vi "Digitizer Analyze_Xout FFT.vi"(7 "Pins":string[](array[string])=["Xout"], 8 "error in":errorcluster, 9 "Published Data Id":string[](array[string]), 10 "Waveform Data In":waveform(dbl)[](array[waveform])=[{"t0"=timestamp(3637030365.2340937 s since 1904-01-01), "dt"=3.3333333333333334e-08, "Y"=array[5343 elements]}, {"t0"=timestamp(3637030365.2340937 s since 1904-01-01), "dt"=3.3333333333333334e-08, "Y"=array[5343 elements]}], 11 "Semiconductor Module Context":T1) -> (0 "error out":errorcluster, 2 "XoutPower":dbl[](array[numeric]), 3 "Xout Frequency":dbl[](array[numeric]))   [LabVIEW 2014]
doc: "Example: Measurement Library\n\nRecommended Input Signal: 100 kHz, 2 Vpp, sine wave\n\nDevices Supported: Refer to NI Example Finders\n\nLabVIEW Description:\n\nThis example illustrates fetching scalar measurements from NI-SCOPE, such as period and rise time calculations. \n\nSome common horizontal and vertical parameters are configured for the oscilloscope. The property node is used to set the reference level units, and the low, middle and high reference levels. For more information about measurement library parameters, see the NI-SCOPE VI Reference Help file. \n\nAfter the Read VI is called to acquire a waveform, the Fetch Measurement Stats VI is used to perform the desired scalar measurement analysis on the waveform. NI-SCOPE keeps a history of each measurement's results, which allows it to retrieve the statistics computed over multiple acquisitions. These statistics include the mean, standard deviation, min, max and number of acquisitions used in the statistics. The statistics are updated once per acquisition when the measurement is fetched. The Clear Stats VI clears this history."
uses:
  <vilib>/NI_TestStand_SemiconductorModule/NI_TestStand_Semiconductor_Module.lvlibp/PinMap/General/SemiconductorModuleContext.ctl
  <vilib>/NI_TestStand_SemiconductorModule/NI_TestStand_Semiconductor_Module.lvlibp/PinMap/General/NIInstrumentTypeIDs.ctl
  <vilib>/measure/matone.llb/Extract Single Tone Information 1 Chan.vi
  <vilib>/NI_TestStand_SemiconductorModule/NI_TestStand_Semiconductor_Module.lvlibp/PinMap/General/Publish/PublishDataDoubleFunctionalTest.vi
  <vilib>/NI_TestStand_SemiconductorModule/NI_TestStand_Semiconductor_Module.lvlibp
  <vilib>/measure/NI_MAPro.lvlib
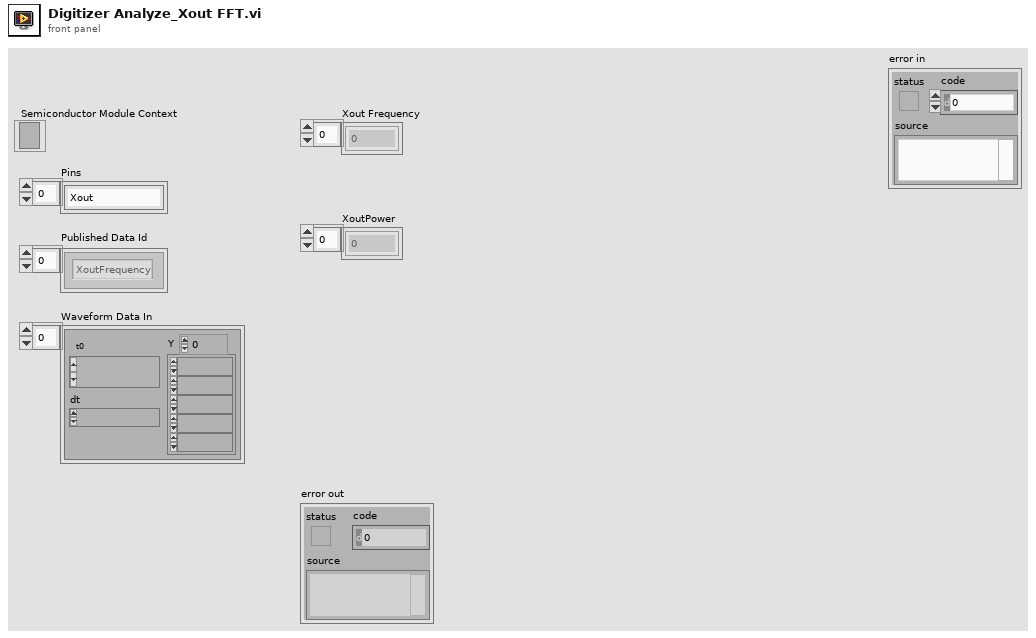
[diagram p1: front panel]
types:
  T1 = typedef "NI_TestStand_Semiconductor_Module.lvlibp/SemiconductorModuleContext.ctl" = refnum<k7>
  T2 = typedef "NI_TestStand_Semiconductor_Module.lvlibp/NIInstrumentTypeIDs.ctl" = string
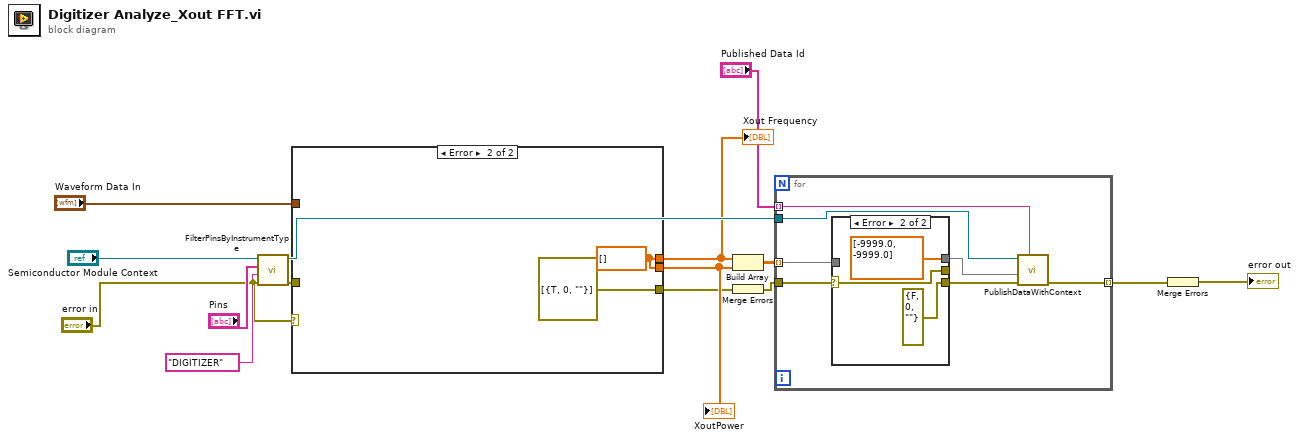
[diagram p0: block diagram]
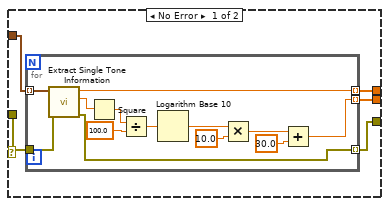
[diagram p2: hidden frame]
diagram:
  n1 = call <vilib>:"FilterPinsByInstrumentType.vi"("error in (no error)"="error in", "Instrument Type Id"=T2 "DIGITIZER", "Pins"="Pins", "Semiconductor Module Context"="Semiconductor Module Context") -> ("error out"=w9:errorcluster, "Semiconductor Module Context Out"=w10:T1)  [unwired: 5 in, 1 out]
  n2 = case shown="Error" "error in" {
    tunnel: "Waveform Data In" -> [w20 _]
    tunnel: w9 -> [w19 _]
    tunnel: [w18 w35] -> w8
    tunnel: [w17 w35] -> w7
    tunnel: [w16 errorcluster[] [{"status"=TRUE, "code"=0, "source"=""}]] -> w4
    frame No Error {
      n3 = for {
        tunnel: w20 -> [w33] mode=indexing
        tunnel: [w32] -> w18 mode=indexing
        tunnel: [w21] -> w17 mode=indexing
        tunnel: w19 -> [w31]
        tunnel: [w30] -> w16 mode=indexing
        n4 = call-poly <vilib>:"Extract Single Tone Information.vi"("error in (no error)"=w31, "time signal in"=w33) -> ("error out"=w30:errorcluster, "detected amplitude"=w29:dbl, "detected frequency"=w32:dbl)  [unwired: 4 in, 3 out]
        n5 = Square(x=w29) -> (x^2=w28:dbl)
        n6 = Divide(x=w28, y=100.0) -> (x/y=w26:dbl)
        n7 = Logarithm Base 10(1:w26) -> (0:w25:dbl)
        n8 = Multiply(x=w25, y=10.0) -> (x*y=w23:dbl)
        n9 = Add(x=w23, y=30.0 ("x*y")) -> (x+y=w21:dbl)
      }
    }
    frame Error {
      w35 = dbl[] []
    }
  }
  "Xout Frequency" <- w8
  "XoutPower" <- w7
  n10 = Build Array(w8, w7) -> (w6:dbl[][])
  n11 = Merge Errors(w4) -> (w3:errorcluster)
  n12 = for {
    tunnel: "Published Data Id" -> [w41] mode=indexing
    tunnel: w10 -> [w40]
    tunnel: w6 -> [w39] mode=indexing
    tunnel: w3 -> [w37]
    tunnel: [w42] -> w13 mode=indexing
    n13 = case shown="Error" w37 {
      selector: w37 -> [w44 w46]
      tunnel: [w43 dbl[] [-9999.0, -9999.0]] -> w36
      tunnel: [w44 errorcluster {"status"=FALSE, "code"=0, "source"=""} ("error IO")] -> w38
      tunnel: [w44 w46] -> _
      tunnel: w39 -> [w43 _]
      frame No Error {
      }
      frame Error {
      }
    }
    n14 = call-poly <vilib>:"PublishDataWithContext.vi"("Published Data Id"=w41, "error in (no error)"=w38, "Data In"=w36, "Semiconductor Module Context"=w40) -> ("error out"=w42:errorcluster)  [unwired: 6 in, 1 out]
  }
  n15 = Merge Errors(w13) -> (→"error out":errorcluster)
